vi "Main.vi"() -> ()   [LabVIEW 2021]
doc: "The myRIO Project template acquires acceleration data from the onboard accelerometer and displays the changes of acceleration values in a waveform chart."
uses:
  <vilib>/myRIO/Express VI/Onboard IO/UART/UART Express VI.xnode
  <vilib>/myRIO/Instrument Drivers/Onboard IO/UART/typedef/VISA Configuration.ctl
  <vilib>/myRIO/Instrument Drivers/Onboard IO/UART/UART.lvlib
  <vilib>/Instr/_visa.llb/VISA Configure Serial Port (Instr).vi
  <vilib>/Utility/file.llb/Write Delimited Spreadsheet (DBL).vi
  <vilib>/myRIO/Express VI/Onboard IO/Encoder/Encoder Express VI.xnode
  <vilib>/myRIO/Instrument Drivers/Onboard IO/Encoder/vis/Read.vi
  <vilib>/myRIO/Instrument Drivers/Onboard IO/Encoder/Encoder.lvlib
  <vilib>/myRIO/Common/Instrument Driver Framework/myRIO v1.0/Encoder/typedefs/Encoder Signal Mode.ctl
  <vilib>/myRIO/Common/Instrument Driver Framework/myRIO v1.0/Encoder/typedefs/Encoder Channels Enum.ctl
  <vilib>/myRIO/Common/Instrument Driver Framework/Utilities/typedefs/Generic FPGA Reference.ctl
  <vilib>/myRIO/Common/Instrument Driver Framework/Utilities/typedefs/myRIO v1.0 Reference.ctl
  <vilib>/myRIO/Common/Instrument Driver Framework/Utilities/typedefs/Hardware Version Enum.ctl
  <vilib>/myRIO/Common/Instrument Driver Framework/Utilities/typedefs/myRIO Generic Hardware Reference.ctl
  <vilib>/myRIO/Instrument Drivers/Onboard IO/Encoder/typedefs/Encoder Reference.ctl
  <vilib>/myRIO/Instrument Drivers/Onboard IO/Encoder/vis/myRIO Encoder Open.xnode
  <vilib>/myRIO/Common/Instrument Driver Framework/Utilities/vis/Is FPGA Ref Available.vi
  <vilib>/myRIO/Common/Instrument Driver Framework/myRIO v1.0/Encoder/vis/myRIO v1.1 Open Encoder.vi
  <vilib>/myRIO/Common/Instrument Driver Framework/myRIO v1.0/Encoder/vis/myRIO v1.0 Configure Encoder.vi
  <vilib>/myRIO/Common/Instrument Driver Framework/myRIO v1.0/Encoder/typedefs/Encoder Configuration v1.0.ctl
  <vilib>/userDefined/High Color/nirio_resource_hc.ctl
  <vilib>/myRIO/Express VI/Onboard IO/PWM/PWM Express VI.xnode
  <vilib>/myRIO/Instrument Drivers/Onboard IO/PWM/vis/Set Duty Cycle and Frequency.vi
  <vilib>/myRIO/Instrument Drivers/Onboard IO/PWM/PWM.lvlib
  <vilib>/myRIO/Instrument Drivers/Onboard IO/PWM/typedefs/PWM Configuration.ctl
  <vilib>/myRIO/Common/Instrument Driver Framework/myRIO v1.0/PWM/typedefs/PWM Channels Enum.ctl
  <vilib>/myRIO/Instrument Drivers/Onboard IO/PWM/typedefs/PWM Reference.ctl
  <vilib>/myRIO/Instrument Drivers/Onboard IO/PWM/vis/myRIO PWM Open.xnode
  <vilib>/myRIO/Common/Instrument Driver Framework/myRIO v1.0/PWM/vis/myRIO v1.1 Open PWM.vi
  <vilib>/myRIO/Instrument Drivers/Utilities/Utilities.lvlib
panel:
  out "Cluster Target":i32[](array[numeric])
  out "Cluster Center":i32[](array[numeric])
  out "Encoder Value":i32
  out "MODE":string
  out "Voltage Out":ext
  in  "Voltage Mapping":ext[](array[numeric])
  in  "Distance Mapping":ext[](array[numeric])
  out "Distance to Detection (ft)":string
  out "Image Out 2":T1(plugin-control)
  out "Z":dbl
  out "Y":dbl
  out "X":dbl
  in  "START":bool caption="Stop (F)"
  out "Orientation":string
  in  "STOP":bool caption="Stop (F)"
  out "Image Out":T1(plugin-control)
  # "defaults for distance\n1: -4.441002452060697 \n2: 22.556228308181506\ndefaults for voltage\n1: 1.14\n2: 0.05"
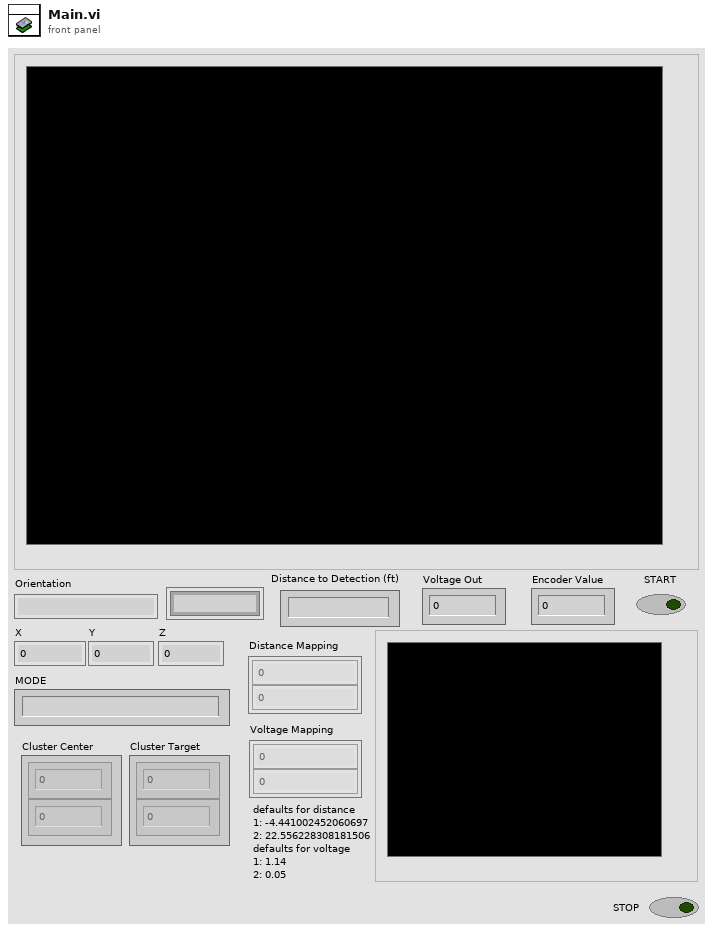
[diagram p1: front panel]
types:
  T1 = typedef "IMAQ Image.ctl" = refnum<image>
  T2 = typedef "PWM.lvlib/PWM Reference.ctl" = cluster{"myRIO Reference":T3, "PWM Channels Enum":T7, "PWM Configuration":T8}
  T3 = typedef "myRIO Generic Hardware Reference.ctl" = cluster{"myRIO Model":T4, "myRIO Hardware Reference":T5}
  T4 = typedef "Hardware Version Enum.ctl" = enum16{"Unknown", "myRIO-1900", "myRIO-1950", "roboRIO", "NI ELVIS RIO CM", "ELVIS III"}
  T5 = typedef "myRIO v1.0 Reference.ctl" = cluster{"Generic FPGA Reference":T6, "Allow multiple opens":bool}
  T6 = typedef "Generic FPGA Reference.ctl" = refnum<k20>
  T7 = typedef "PWM Channels Enum.ctl" = enum16{"Not Connected", "C/PWM0", "C/PWM1", "A/PWM0", "A/PWM1", "A/PWM2", "A/PWM3", "A/PWM4", "A/PWM5", "A/PWM6", "A/PWM7", "A/PWM8", "A/PWM9", "A/PWM10", "A/PWM11", "A/PWM12", "A/PWM13", "A/PWM14", "A/PWM15", "A/PWM16", "A/PWM17", "A/PWM18", "A/PWM19", "B/PWM0", "B/PWM1", "B/PWM2", "B/PWM3", "B/PWM4", "B/PWM5", "B/PWM6", "B/PWM7", "B/PWM8", "B/PWM9", "B/PWM10", "B/PWM11", "B/PWM12", "B/PWM13", "B/PWM14", "B/PWM15", "B/PWM16", "B/PWM17", "B/PWM18", "B/PWM19", "PWM/PWM0", "PWM/PWM1", "PWM/PWM2", "PWM/PWM3", "PWM/PWM4", "PWM/PWM5", "PWM/PWM6", "PWM/PWM7", "PWM/PWM8", "PWM/PWM9"}
  T8 = typedef "PWM.lvlib/PWM Configuration.ctl" = cluster{"Frequency":dbl, "Duty Cycle":dbl}
  T9 = typedef "nirio_resource_hc.ctl" = tag
  T10 = typedef "Encoder.lvlib/Encoder Reference.ctl" = cluster{"myRIO Reference":T3, "Encoder Channels Enum":T11}
  T11 = typedef "Encoder Channels Enum.ctl" = enum16{"Not Connected", "C/ENC0", "C/ENC1", "A/ENC", "A/ENC0", "A/ENC1", "A/ENC2", "A/ENC3", "A/ENC4", "A/ENC5", "A/ENC6", "A/ENC7", "A/ENC8", "A/ENC9", "B/ENC", "B/ENC0", "B/ENC1", "B/ENC2", "B/ENC3", "B/ENC4", "B/ENC5", "B/ENC6", "B/ENC7", "B/ENC8", "B/ENC9", "DIO/ENC0", "DIO/ENC1", "DIO/ENC2", "DIO/ENC3", "DIO/ENC4"}
  T12 = typedef "Encoder Signal Mode.ctl" = enum16{"Quadrature phase signal", "Step and direction signal"}
  T13 = typedef "UART.lvlib/VISA Configuration.ctl" = cluster{"baud rate (9600)":u32, "data bits (8)":u16, "parity (0:none)":enum16{"None", "Odd", "Even", "Mark", "Space"}, "stop bits (10: 1 bit)":u16, "flow control (0:none)":u16, "termination char\n(0xA = '\\n' = LF) ":u8, "Enable Termination\nChar (T)":bool, "timeout (10sec)":u32}
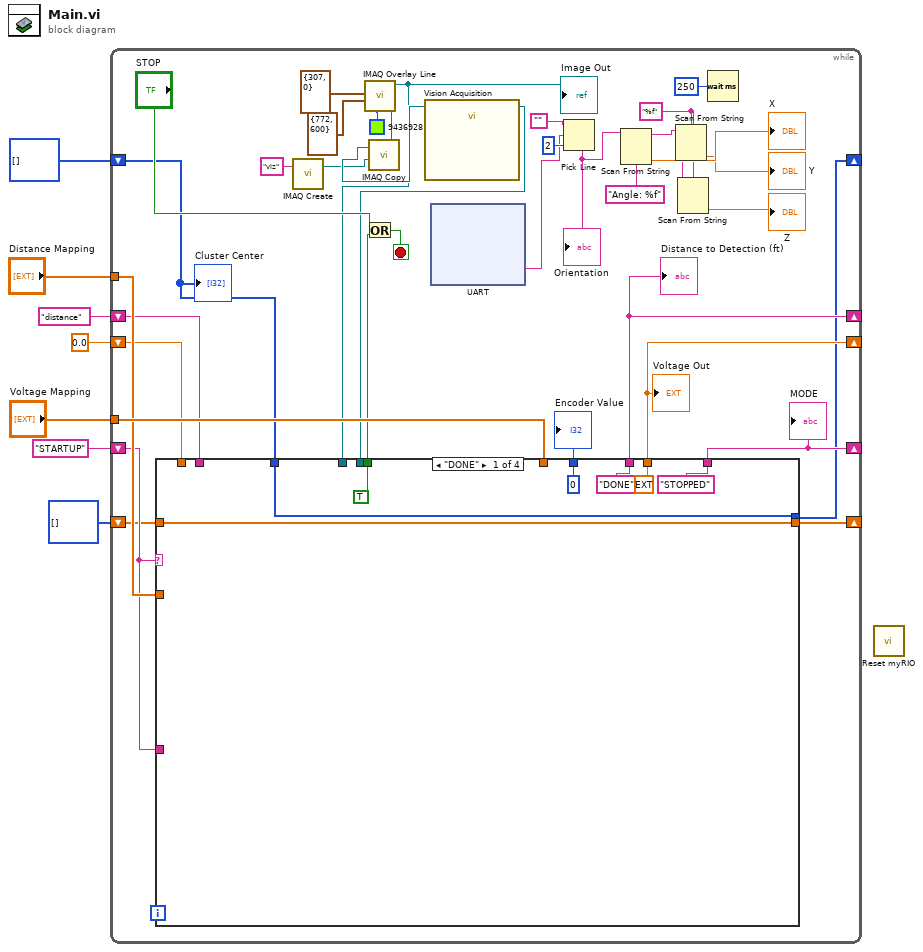
[diagram p0: block diagram]
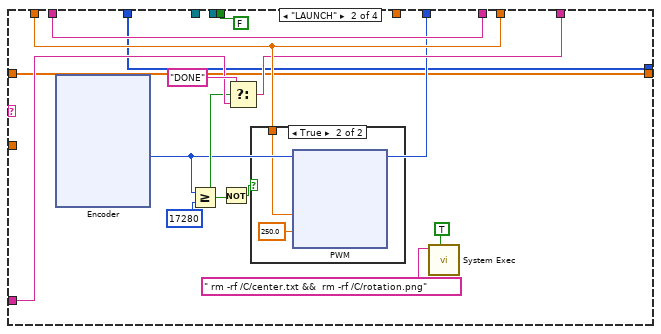
[diagram p2: hidden frame]
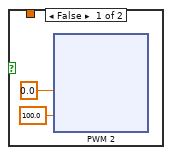
[diagram p3: hidden frame]
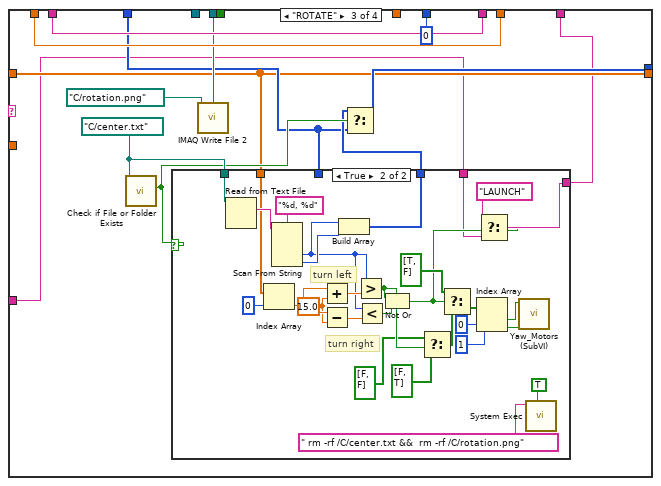
[diagram p4: hidden frame]
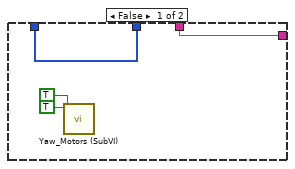
[diagram p5: hidden frame]
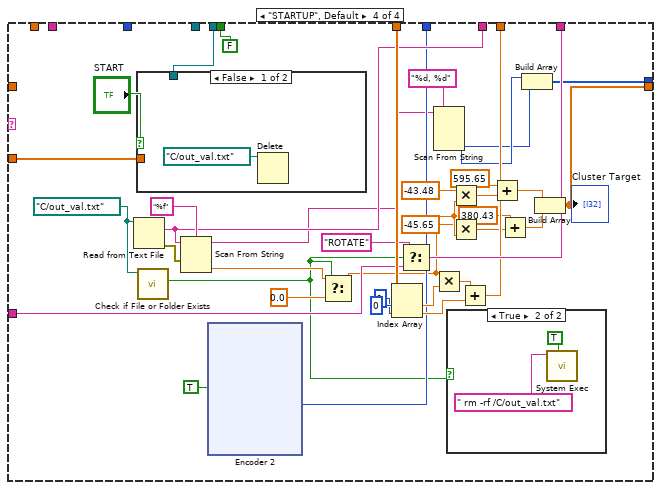
[diagram p6: hidden frame]
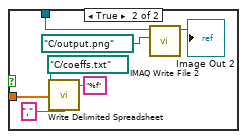
[diagram p8: hidden frame]
diagram:
  n1 = while {
    tunnel: "Distance Mapping" -> [w30]
    shift-right: [w29] -> _
    shift-left: "STARTUP" -> [w15]
    tunnel: "Voltage Mapping" -> [w31]
    shift-right: [w25] -> _
    shift-left: 0.0 -> [w26]
    shift-right: [w27] -> _
    shift-left: "distance" -> [w28]
    shift-right: [w14] -> _
    shift-left: i32[] [] -> [w13]
    shift-right: [w10] -> _
    shift-left: i32[] [] -> [w9]
    stop <- w22 stop-if-true
    w36 = "%f" ("format string")
    n2 = call "IMAQ Create"("Image Name"="viz") -> ("New Image"=w17:T1)  [unwired: 4 in, 1 out]
    n3 = call "Vision Acquisition"() -> ("Image Out"=w18:T1)  [unwired: 25 in, 2 out]
    n4 = call "IMAQ Copy"("Image Dst"=w17, "Image Src"=w18) -> ("Image Dst Out"=w19:T1)  [unwired: 4 in, 1 out]
    n5 = call "IMAQ Overlay Line"("Color"=u32 9436928, "End Point"=cluster{"X":i32, "Y":i32} {"X"=772, "Y"=600}, "Start Point"=cluster{"X":i32, "Y":i32} {"X"=307, "Y"=0}, "Image"=w19) -> ("Image Out"=w8:T1)  [unwired: 6 in, 1 out]
    "Image Out" <- w8
    n6 = case shown="\"DONE\"" w15 {
      tunnel: w31 -> [_ _ _ w262]
      tunnel: w15 -> [_ w60 w185 w259]
      tunnel: w18 -> [_ _ w194 w255]
      tunnel: w30 -> [_ _ _ w254]
      tunnel: ["STOPPED" w59 w186 w253] -> w29
      tunnel: w26 -> [_ w62 w196 _]
      tunnel: w28 -> [_ w64 w197 _]
      tunnel: ["DONE" w64 w197 w251] -> w27
      tunnel: [ext 0.0 w62 w196 w252] -> w25
      tunnel: [TRUE FALSE _ FALSE] -> w24
      tunnel: [0 ("Counter Value") w55 0 ("Counter Value") w248] -> w21
      tunnel: [w45 w54 w189 w243] -> w14
      tunnel: w13 -> [w45 w54 w188 _]
      tunnel: [w44 w53 w187 w231] -> w10
      tunnel: w9 -> [w44 w53 w187 _]
      tunnel: w8 -> [_ _ _ _]
      frame "DONE" {
      }
      frame "LAUNCH" {
        n7 = xnode "Encoder"() -> ("Counter Value"=w55:i32)  [unwired: 2 in, 3 out]
        n8 = Greater Or Equal?(x=w55, y=17280) -> (x >= y?=w57:bool)
        n9 = Not(x=w57) -> (.not. x?=w56:bool)
        n10 = Select(t="DONE", s=w57, f=w60) -> (s? t:f=w59:string)
        n11 = case shown="True" w56 {
          tunnel: w62 -> [_ w103]
          frame False {
            n12 = xnode "PWM 2"("Duty Cycle"=0.0, "Frequency [Hz]"=100.0) -> ()  [unwired: 1 in, 1 out]
          }
          frame True {
            n13 = xnode "PWM"("Duty Cycle"=w103, "Frequency [Hz]"=250.0) -> ()  [unwired: 1 in, 1 out]
          }
        }
        n14 = call <vilib>:"System Exec.vi"("wait until completion? (T)"=TRUE, "command line"=" rm -rf /C/center.txt &&  rm -rf /C/rotation.png") -> ()  [unwired: 6 in, 4 out]
      }
      frame "ROTATE" {
        w192 = path "C:/center.txt" ("File Path")
        n15 = call <vilib>:"Check if File or Folder Exists.vi"("path"=w192) -> ("file or folder exists?"=w191:bool)  [unwired: 8 in, 2 out]
        n16 = case shown="True" w191 {
          tunnel: w192 -> [_ w229]
          tunnel: [w201 w226] -> w190
          tunnel: w188 -> [w201 _]
          tunnel: w187 -> [_ w225]
          tunnel: [w200 w209] -> w186
          tunnel: w185 -> [w200 w207]
          frame False {
            n17 = call "Yaw_Motors (SubVI).vi"("POWER"=TRUE, "DIR"=TRUE) -> ()  [unwired: 10 in]
          }
          frame True {
            w202 = 15.0 ("y")
            # "turn right"
            # "turn left"
            n18 = Read from Text File(file (use dialog)=w229) -> (text=w230:string)  [unwired: 3 in, 3 out]
            n19 = Index Array(array=w225, index=0) -> (element=w203:dbl)
            n20 = Scan From String(format string="%d, %d", input string=w230) -> (output 1=w221:i32, output 2=w227:i32)  [unwired: 4 in, 3 out]
            n21 = Add(x=w203, y=w202) -> (x+y=w223:dbl)
            n22 = Subtract(x=w203, y=w202) -> (x-y=w222:dbl)
            n23 = Build Array(w221, w227) -> (w226:i32[])
            n24 = Greater?(x=w221, y=w223) -> (0:w218:bool)
            n25 = Less?(x=w221, y=w222) -> (x < y?=w220:bool)
            n26 = Not Or(1:w220, 2:w218) -> (0:w208:bool)
            n27 = Select(t=bool[] [FALSE, FALSE], s=w218, f=bool[] [FALSE, TRUE]) -> (s? t:f=w217:bool[])
            n28 = Select(t=bool[] [TRUE, FALSE], s=w208, f=w217) -> (s? t:f=w214:bool[])
            n29 = Index Array(array=w214, index #1=0 ("index"), index #2=1 ("index")) -> (element #1=w211:bool, element #2=w210:bool)
            n30 = Select(t="LAUNCH", s=w208, f=w207) -> (s? t:f=w209:string)
            n31 = call "Yaw_Motors (SubVI).vi"("POWER"=w210, "DIR"=w211) -> ()  [unwired: 10 in]
            n32 = call <vilib>:"System Exec.vi"("wait until completion? (T)"=TRUE, "command line"=" rm -rf /C/center.txt &&  rm -rf /C/rotation.png") -> ()  [unwired: 6 in, 4 out]
          }
        }
        n33 = call-poly "IMAQ Write File 2"("File Path"=path "C:/rotation.png", "Image"=w194) -> ()  [unwired: 8 in, 2 out]
        n34 = Select(t=w190, s=w191, f=w188) -> (s? t:f=w189:i32[])
      }
      frame "STARTUP", Default {
        w247 = path "C:/out_val.txt" ("file path (use dialog)")
        n35 = Read from Text File(file (use dialog)=w247) -> (text=w251:string, error out=w264:errorcluster)  [unwired: 3 in, 2 out]
        n36 = case shown="False" "START" {
          tunnel: w255 -> [_ w324]
          tunnel: w254 -> [_ w318]
          frame False {
            n37 = Delete(path (use dialog)=path "C:/out_val.txt") -> ()  [unwired: 4 in, 3 out]
          }
          frame True {
            n38 = call-poly <vilib>:"Write Delimited Spreadsheet.vi"("file path (dialog if empty)"=path "C:/coeffs.txt", "format (%.3f)"="%f", "1D data"=w318, "delimiter (\\t)"="," ("delimiter (\\t)")) -> ()  [unwired: 10 in, 2 out]
            n39 = call-poly "IMAQ Write File 2"("File Path"=path "C:/output.png", "Image"=w324) -> ("Image Out (duplicate)"=→"Image Out 2":T1)  [unwired: 8 in, 1 out]
          }
        }
        n40 = call <vilib>:"Check if File or Folder Exists.vi"("path"=w247) -> ("file or folder exists?"=w246:bool)  [unwired: 8 in, 2 out]
        n41 = Scan From String(format string="%f", input string=w251, error in=w264) -> (remaining string=w245:string, output 1=w265:dbl)  [unwired: 2 in, 2 out]
        n42 = xnode "Encoder 2"("Reset Counter"=TRUE) -> ("Counter Value"=w248:i32)  [unwired: 1 in, 3 out]
        n43 = Select(t=w265, s=w246, f=0.0) -> (s? t:f=w240:dbl)
        n44 = Index Array(array=w262, index #1=0 ("index"), index #2=1 ("index")) -> (element #1=w266:ext, element #2=w268:ext)
        n45 = Select(t="ROTATE", s=w246, f=w259) -> (s? t:f=w253:string)
        n46 = Scan From String(format string="%d, %d", input string=w245) -> (output 1=w244:i32, output 2=w241:i32)  [unwired: 4 in, 3 out]
        n47 = Multiply(x=w240, y=w266) -> (x*y=w267:ext)
        n48 = case shown="True" w246 {
          frame False {
          }
          frame True {
            n49 = call <vilib>:"System Exec.vi"("wait until completion? (T)"=TRUE, "command line"=" rm -rf /C/out_val.txt") -> ()  [unwired: 6 in, 4 out]
          }
        }
        n50 = Multiply(x=-43.48, y=w240) -> (x*y=w237:dbl)
        n51 = Multiply(x=-45.65, y=w240) -> (x*y=w234:dbl)
        n52 = Add(x=w267, y=w268) -> (x+y=w252:ext)
        n53 = Add(x=595.65, y=w237) -> (x+y=w233:dbl)
        n54 = Add(x=380.43, y=w234) -> (x+y=w232:dbl)
        n55 = Build Array(w244, w241) -> (w243:i32[])
        n56 = Build Array(w233, w232) -> (w231:dbl[])
        "Cluster Target" <- w231
      }
    }
    "Distance to Detection (ft)" <- w27
    "Voltage Out" <- w25
    "MODE" <- w29
    "Encoder Value" <- w21
    n57 = Or(x="STOP", y=w24) -> (x .or. y?=w22:bool)
    n58 = xnode "UART"() -> ("Characters Read"=w40:string)  [unwired: 1 in, 1 out]
    n59 = Pick Line(string ("")="", multi-line string=w40, line index=2) -> (output string=w39:string)
    "Orientation" <- w39
    n60 = Scan From String(format string="Angle: %f", input string=w39) -> (remaining string=w32:string, output 1=→"X":dbl)  [unwired: 3 in, 2 out]
    n61 = Scan From String(format string=w36, input string=w32) -> (remaining string=w35:string, output 1=→"Y":dbl)  [unwired: 3 in, 2 out]
    n62 = Scan From String(format string=w36, input string=w35) -> (output 1=→"Z":dbl)  [unwired: 3 in, 3 out]
    n63 = Wait (ms)(milliseconds to wait=u32 250) -> ()  [unwired: 1 out]
    "Cluster Center" <- w13
  }
  n64 = call <vilib>:"Reset myRIO.vi"() -> ()  [unwired: 11 in, 1 out]
